vi "readKeysFromConfigFile.vi"(8 "error in (no error)":errorcluster, 9 "key":string, 10 "section":string, 11 "Refnum in":T1) -> (0 "error out":errorcluster, 2 "arrayOfKeys":string[](array[string]), 3 "Refnum out":T1)   [LabVIEW 2018]
doc: "Read the keys of one section in INI file and put them in an array of keys.\n\nNOTE: this is only for internal use. User does not call this function directly."
uses:
  <vilib>/Utility/config.llb/Config Data RefNum.ctl
  <vilib>/Utility/config.llb/Read Key (String).vi
  <vilib>/Utility/config.llb/NI_LVConfig.lvlib
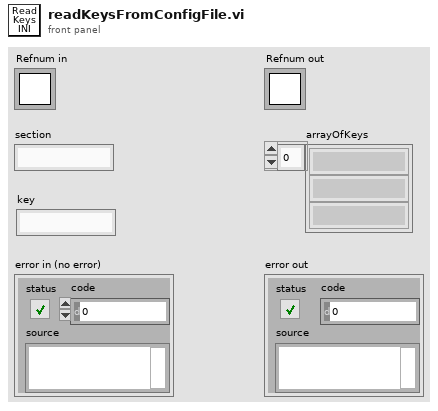
[diagram p1: front panel]
types:
  T1 = typedef "NI_LVConfig.lvlib/Config Data RefNum.ctl" = refnum<k1>
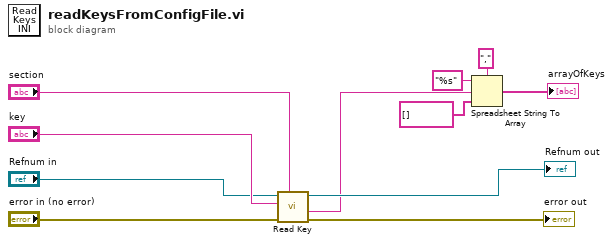
[diagram p0: block diagram]
diagram:
  n1 = call-poly <vilib>:"Read Key.vi"("section"="section", "error in (no error)"="error in (no error)", "key"="key", "refnum"="Refnum in") -> ("error out"=→"error out":errorcluster, "value"=w2:string, "refnum out"=→"Refnum out":T1)  [unwired: 4 in, 1 out]
  n2 = Spreadsheet String To Array(delimiter (Tab)=",", format string="%s", spreadsheet string=w2, array type (2D Dbl)=string[] [] ("value")) -> (array=→"arrayOfKeys":string[])
